vi "Run.vi"(6 "Type Y":T2(ring), 7 "Type X":T2(ring), 8 "error in (no error)":errorcluster caption="entrée d'erreur (pas d'erreur)", 9 "Y":string[][](array[string]), 10 "X":string[][](array[string]), 11 "Euclidean_distances.lvclass":refnum<class "Euclidean_distances.lvclass">) -> (0 "error out":errorcluster caption="sortie d'erreur", 2 "Data":T1, 3 "Euclidean_distances.lvclass":refnum<class "Euclidean_distances.lvclass">)   [LabVIEW 2020, in "Euclidean_distances.lvclass"]
doc: "Returns : \n\n- distances : array, shape (n_samples_1, n_samples_2)"
uses:
  Euclidean_distances.lvclass
  Euclidean_distances.lvclass/Euclidean_distances.ctl
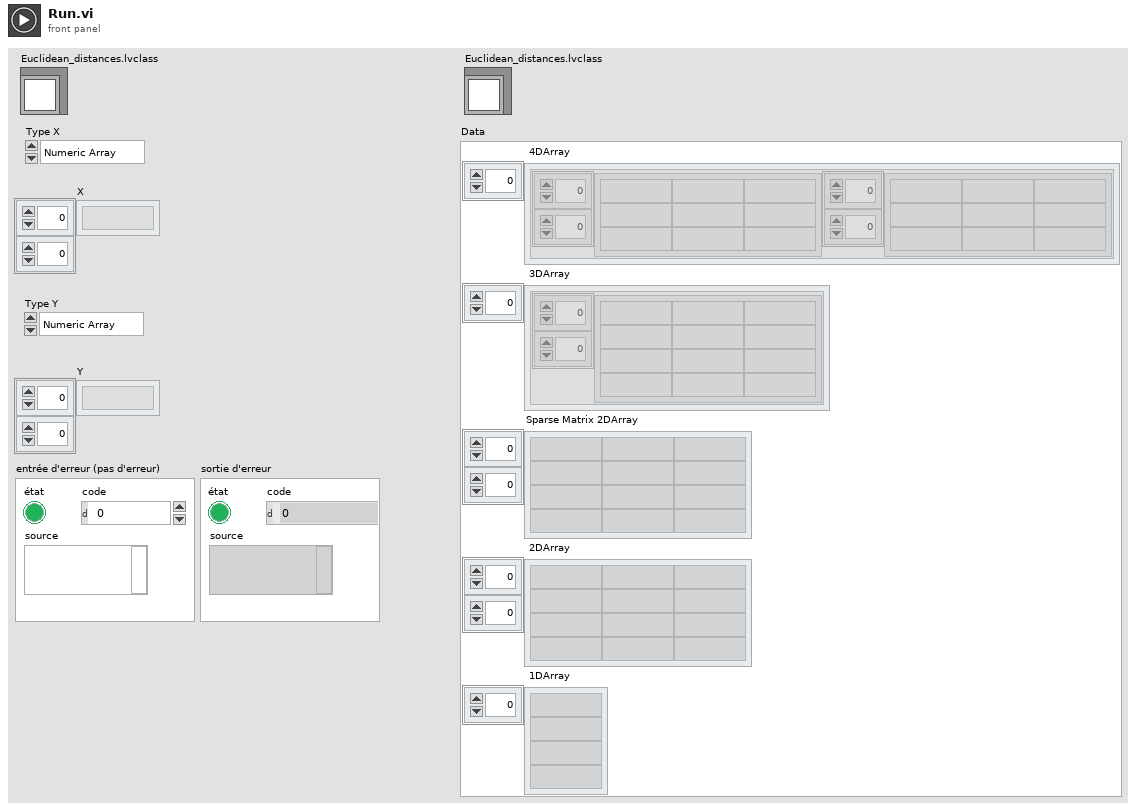
[diagram p1: front panel]
types:
  T1 = cluster{" 4DArray":cluster{"1":string[][], "2":string[][]}[], " 3DArray":cluster{"Tableau":string[][]}[], "Sparse Matrix 2DArray":string[][], " 2DArray":string[][], " 1DArray":string[]}
  T2 = enum16{"Numeric Array", "String Array", "Sparse"}
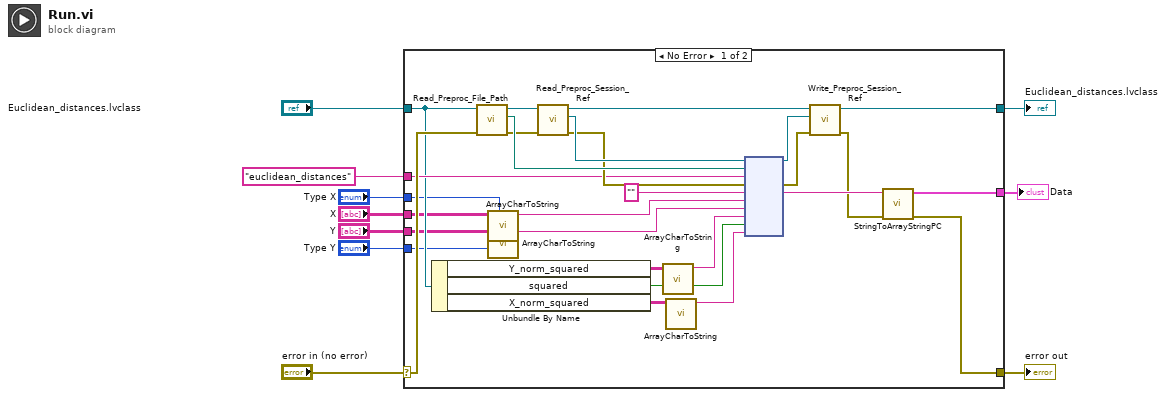
[diagram p0: block diagram]
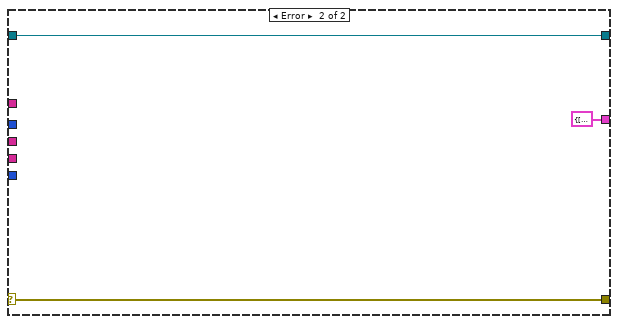
[diagram p2: hidden frame]
diagram:
  n1 = case shown="No Error" "error in (no error)" {
    selector: "error in (no error)" -> [w29 w41]
    tunnel: [w12 w41] -> w9
    tunnel: [w15 w40] -> w7
    tunnel: "Euclidean_distances.lvclass" -> [w27 w40]
    tunnel: "euclidean_distances" ("Fonction") -> [w28 _]
    tunnel: "X" -> [w21 _]
    tunnel: "Y" -> [w20 _]
    tunnel: "Type X" -> [w19 _]
    tunnel: "Type Y" -> [w18 _]
    tunnel: [w11 T1 {" 4DArray"=[], " 3DArray"=[], "Sparse Matrix 2DArray"=[], " 2DArray"=[], " 1DArray"=[]} ("Data")] -> w1
    frame No Error {
      n2 = Unbundle By Name(w27) -> ("Y_norm_squared"=w25:string[][], "squared"=w26:bool, "X_norm_squared"=w23:string[][])
      n3 = call-dynamic "Read_Preproc_File_Path.vi"("error in (no error)"=w29, "Python in"=w27) -> ("error out"=w33:errorcluster, "File_Path"=w36:path, "Python out"=w38:refnum<class "Euclidean_distances.lvclass">)  [unwired: 7 in]
      n4 = call "ArrayCharToString.vi"("Type"=w19, "TAB"=w21) -> ("Instruction"=w17:string)  [unwired: 9 in]
      n5 = call "ArrayCharToString.vi"("Type"=w18, "TAB"=w20) -> ("Instruction"=w16:string)  [unwired: 9 in]
      n6 = call-dynamic "Read_Preproc_Session_Ref.vi"("error in (no error)"=w33, "Python in"=w38) -> ("error out"=w34:errorcluster, "Session_ref"=w35:refnum<k35>, "Python out"=w37:refnum<class "Euclidean_distances.lvclass">)  [unwired: 7 in]
      n7 = call "ArrayCharToString.vi"("TAB"=w25) -> ("Instruction"=w24:string)  [unwired: 10 in]
      n8 = call "ArrayCharToString.vi"("TAB"=w23) -> ("Instruction"=w22:string)  [unwired: 10 in]
      n9 = node(w35, w36, w28, w34, "", w17, w16, w24, w26, w22) -> (w30:refnum<k35>, w32:errorcluster, w14:string)  [unwired: 5 in, 2 out]
      n10 = call-dynamic "Write_Preproc_Session_Ref.vi"("error in (no error)"=w32, "Session_ref"=w30, "Python in"=w37) -> ("error out"=w13:errorcluster, "Python out"=w15:refnum<class "Euclidean_distances.lvclass">)  [unwired: 7 in]
      n11 = call "StringToArrayStringPC.vi"("sortie d'erreur"=w13, "Return value"=w14) -> ("sortie d'erreur"=w12:errorcluster, "Data"=w11:T1)  [unwired: 8 in]
    }
    frame Error {
    }
  }
  "error out" <- w9
  "Euclidean_distances.lvclass" <- w7
  "Data" <- w1
